vi "Write Range UI.vi"(8 "error in (no error)":errorcluster, 10 "Set UI to input? (F)":bool, 11 "Scanner in":refnum<class "Scanner.lvclass">) -> (0 "error out":errorcluster, 3 "Scanner out":refnum<class "Scanner.lvclass">)   [LabVIEW 2009, in "Scanner.lvclass"]
doc: "A Setup UI method for the superclass \"Range\" of scanner."
uses:
  Scanner.lvclass
  Scanner.lvclass/Scanner.ctl
  Range.ctl
panel:
  in  "Return to start?":bool
  out "Time Estimate":string
  out "# Points":u32
  in  "Last":dbl
  in  "Step Size":dbl=1.0 min=0.0
  in  "First":dbl
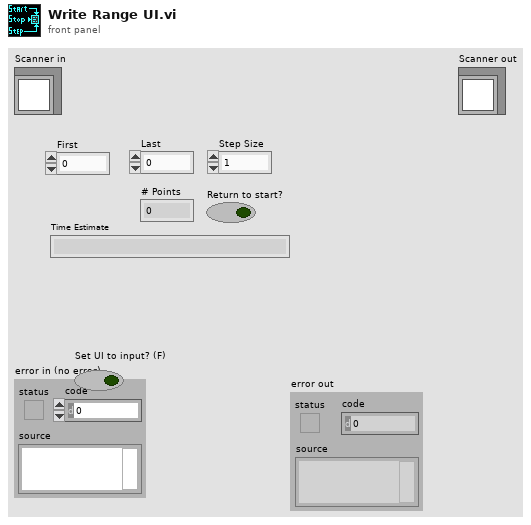
[diagram p1: front panel]
types:
  T1 = typedef "Scanner.lvclass/Range.ctl" = cluster{"xi":dbl, "xf":dbl, "dx":dbl, "Return to start?":bool}
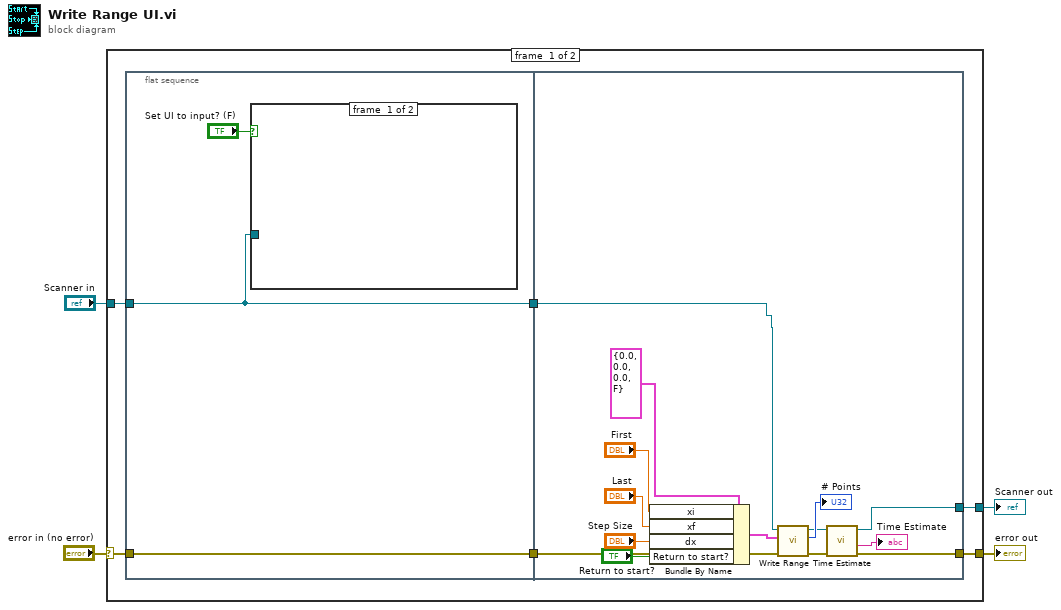
[diagram p0: block diagram]
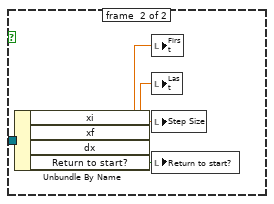
[diagram p2: hidden frame]
diagram:
  n1 = case shown="No Error" "error in (no error)" {
    selector: "error in (no error)" -> [w9 w34]
    tunnel: [w7 w34] -> w3
    tunnel: [w8 w33] -> w1
    tunnel: "Scanner in" -> [w10 w33]
    frame #0 {
      n2 = flat-sequence {
        tunnel: w9 -> [w13]
        tunnel: w10 -> [w11]
        tunnel: [w11] -> w6
        tunnel: [w13] -> w5
        tunnel: [w30] -> w8
        tunnel: [w29] -> w7
        tunnel: w6 -> [w19]
        tunnel: w5 -> [w32]
        frame #0 {
          n3 = case shown="True" "Set UI to input? (F)" {
            tunnel: w11 -> [_ w18]
            frame #0 {
            }
            frame #1 {
              n4 = Unbundle By Name(w18) -> ("xi"=w16:dbl, "xf"=w15:dbl, "dx"=w17:dbl, "Return to start?"=w14:bool)
              n5 = local write "First"(w16) -> ()
              n6 = local write "Last"(w15) -> ()
              n7 = local write "Step Size"(w17) -> ()
              n8 = local write "Return to start?"(w14) -> ()
            }
          }
        }
        frame #1 {
          n9 = Bundle By Name(cluster=T1 {"xi"=0.0, "xf"=0.0, "dx"=0.0, "Return to start?"=FALSE} ("Range"), "xi"="First", "xf"="Last", "dx"="Step Size", "Return to start?"="Return to start?") -> (w25:T1)
          n10 = call-dynamic "Write Range.vi"("error in (no error)"=w32, "Range"=w25, "Scanner in"=w19) -> ("error out"=w26:errorcluster, "# Points"=→"# Points":u32, "Scanner out"=w27:refnum<class "Scanner.lvclass">)  [unwired: 3 in, 3 out]
          n11 = call-dynamic "Time Estimate.vi"("error in (no error)"=w26, "Scanner.lvclass"=w27) -> ("error out"=w29:errorcluster, "Time Estimate"=→"Time Estimate":string, "Scanner.lvclass out"=w30:refnum<class "Scanner.lvclass">)  [unwired: 2 in, 5 out]
        }
      }
    }
    frame #1 {
    }
  }
  "error out" <- w3
  "Scanner out" <- w1
